vi "TCP-Wait For.vi"(0 "Address":string, 5 "Port":i32, 7 "Name":string, 9 "Timeout (ms)":i32=5000, 11 "error in (no error)":errorcluster) -> (15 "error out":errorcluster)   [LabVIEW 2020]
uses:
  Utility VIs/Controls/Utilities-Wait.vi/89bc9713-8f2c-40bd-a11f-1c800a437687.vi
  <vilib>/Utility/High Resolution Polling Wait.vi
  TCP-Prepend String Length.vi
panel:
  in  "milliseconds to wait":u32=100
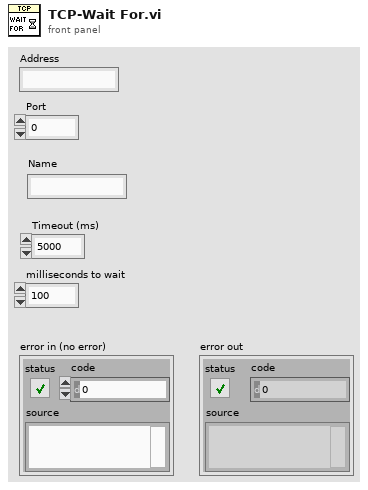
[diagram p1: front panel]
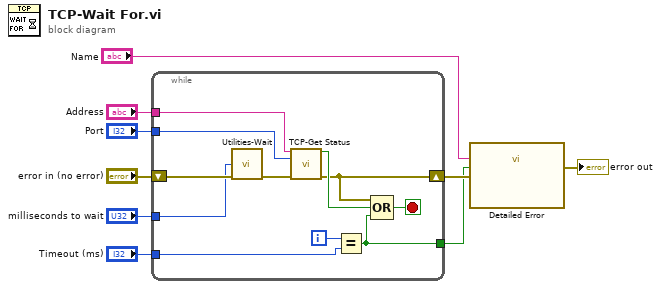
[diagram p0: block diagram]
diagram:
  n1 = while {
    tunnel: "Address" -> [w20]
    tunnel: "Port" -> [w19]
    shift-right: [w16] -> w4
    shift-left: "error in (no error)" -> [w18]
    tunnel: [w13] -> w2
    tunnel: "milliseconds to wait" -> [w11]
    tunnel: "Timeout (ms)" -> [w10]
    i -> [w15]
    stop <- w14 stop-if-true
    n2 = call "Utilities-Wait.vi"("milliseconds to wait"=w11, "error in (no error)"=w18) -> ("error out"=w12:errorcluster)  [unwired: 13 in]
    n3 = call "TCP-Get Status.vi"("IP Address"=w20, "Port"=w19, "error in (no error)"=w12) -> ("status"=w17:bool, "error out"=w16:errorcluster)  [unwired: 11 in]
    n4 = Equal?(x=w15, y=w10) -> (x = y?=w13:bool)
    n5 = Compound Arithmetic op=OR(w16, w17, w13) -> (w14:bool)
  }
  n6 = call "Detailed Error"("Details"="Name", "Error?"=w2, "Primary"=w4) -> ("detailed error"=→"error out":errorcluster)  [unwired: 12 in]
